vi "Experiment Selector.vi"() -> ()   [LabVIEW 2013]
panel:
  in  "Experiment Choices":T1(array[cluster])
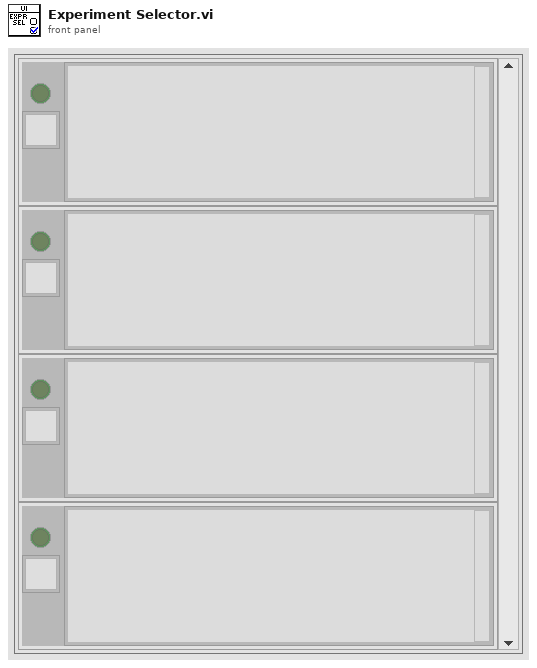
[diagram p1: front panel]
types:
  T1 = cluster{"Selected":bool, "Experimental VI Description":string, "new picture":picture, "Experimental VI Reference":refnum<vi>, "Experimental Data Save VI Reference ":refnum<vi>}[]
  T2 = cluster{bool, "Experimental VI Description":string, "Experimental VI Icon":picture, "Experimental VI Reference":refnum<vi>, "Experimental Data Save VI Reference ":refnum<vi>}
  T3 = cluster{bool, "Experimental VI Description":string, "Experimental VI Icon":picture, "Experimental VI Reference":refnum<vi>, "Experimental Data Save VI Reference ":refnum<vi>}[]
  T4 = cluster{"Selected":bool, "Experimental VI Description":string, "new picture":picture, "Experimental VI Reference":refnum<vi>, "Experimental Data Save VI Reference ":refnum<vi>}
  T5 = typedef "Semaphore RefNum" = refnum<k1>
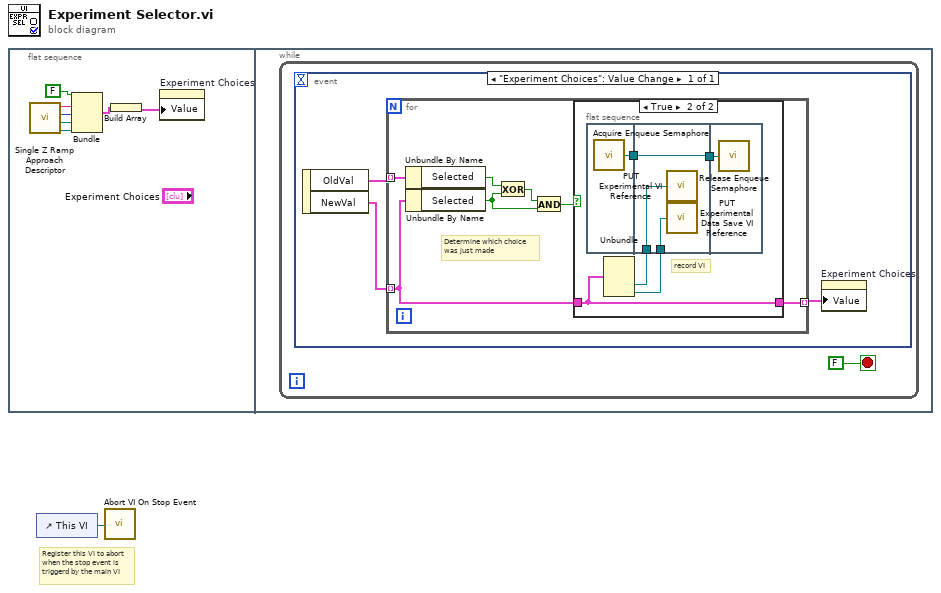
[diagram p0: block diagram]
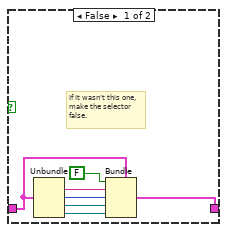
[diagram p2: hidden frame]
diagram:
  # "Register this VI to abort\nwhen the stop event is\ntriggerd by the main VI"
  n1 = flat-sequence {
    frame #0 {
      n2 = call "Single Z Ramp Approach Descriptor.vi"() -> ("Experimental Data Save VI Reference"=w3:refnum<vi>, "Experimental VI Reference"=w4:refnum<vi>, "Experimental VI Icon"=w5:picture, "Experimental VI Description"=w6:string)
      n3 = Bundle(FALSE, "Experimental VI Description"=w6, "Experimental VI Icon"=w5, "Experimental VI Reference"=w4, "Experimental Data Save VI Reference"=w3) -> (w8:T2)  [unwired: 1 in]
      n4 = Build Array(w8) -> (w2:T3)
      n5 = property on="Experiment Choices" class="Arr (strict)"("Value"=w2) -> ()  [unwired: 2 in, 2 out]
    }
    frame #1 {
      n6 = while {
        stop <- FALSE stop-if-true
        n7 = event shown="[0] \"Experiment Choices\": Value Change" {
          selector: _ -> [_]
          dyn-events: _ -> [_]
          timeout: _ -> [_]
          event "Experiment Choices": Value Change {
            n8 = event-data() -> ("OldVal"=w12:T1, "NewVal"=w11:T1)  [unwired: 1 in]
            n9 = for {
              tunnel: w12 -> [w15] mode=indexing
              tunnel: w11 -> [w14] mode=indexing
              tunnel: [w13] -> w10 mode=indexing
              # "Determine which choice\nwas just made"
              n10 = Unbundle By Name(w15) -> ("Selected"=w18:bool)
              n11 = Unbundle By Name(w14) -> ("Selected"=w17:bool)
              n12 = Exclusive Or(1:w17, 2:w18) -> (0:w19:bool)
              n13 = And(x=w19, y=w17) -> (x .and. y?=w16:bool)
              n14 = case shown="True" w16 {
                tunnel: w14 -> [w26 w29]
                tunnel: [w23 w29] -> w13
                frame False {
                  # "If it wasn't this one,\nmake the selector\nfalse."
                  n15 = Unbundle(w26) -> ("Experimental VI Description"=w25:string, "new picture"=w24:picture, "Experimental VI Reference"=w22:refnum<vi>, "Experimental Data Save VI Reference"=w21:refnum<vi>)  [unwired: 1 out]
                  n16 = Bundle(cluster=w26, "Selected"=FALSE, "Experimental VI Description"=w25, "new picture"=w24, "Experimental VI Reference"=w22, "Experimental Data Save VI Reference"=w21) -> (w23:T4)
                }
                frame True {
                  # "record VI"
                  n17 = flat-sequence {
                    tunnel: [w32] -> w31
                    tunnel: w31 -> [w35]
                    tunnel: [w35] -> w30
                    tunnel: w28 -> [w34]
                    tunnel: w27 -> [w33]
                    tunnel: w30 -> [w36]
                    frame #0 {
                      n18 = call "Acquire Enqueue Semaphore.vi"() -> ("Semaphore Reference"=w32:T5)
                    }
                    frame #1 {
                      n19 = call "PUT Experimental VI Reference.vi"("Experimental VI Reference"=w34) -> ()
                      n20 = call "PUT Experimental Data Save VI Reference.vi"("Experimental Data Save VI Reference"=w33) -> ()
                    }
                    frame #2 {
                      n21 = call "Release Enqueue Semaphore.vi"("Semaphore Reference"=w36) -> ()
                    }
                  }
                  n22 = Unbundle(w29) -> ("Experimental VI Reference"=w28:refnum<vi>, "Experimental Data Save VI Reference"=w27:refnum<vi>)  [unwired: 3 out]
                }
              }
            }
            n23 = property on="Experiment Choices" class="Arr (strict)"("Value"=w10) -> ()  [unwired: 2 in, 2 out]
          }
        }
      }
    }
  }
  n24 = control-ref of="This VI"() -> (w1:refnum<vi>)
  n25 = call "Abort VI On Stop Event.vi"("VI Reference"=w1) -> ()
